vi "KE622x -- Set Current Range.vi"(0 "Resource In":refnum<visa-resource-name>, 1 "Check For SCPI Errors? (T)":bool=TRUE, 7 "Current Range In":T1, 11 "error in (no error)":errorcluster, 12 "Read Back Set Values? (T)":bool=TRUE) -> (4 "Resource Out (dupl)":refnum<visa-resource-name>, 8 "Current Range Out":T1, 15 "error out":errorcluster)   [LabVIEW 2020, in "Keithley 622x.lvlib"]
doc: "Allows the user to either auto-select the current range based on the current level, or manually specify a range."
uses:
  Keithley 622x.lvlib
  Typedefs/KE622x -- Current Ranges.ctl
  C/Program Files/National Instruments/LabVIEW 2021/instr.lib/Keithley 622x LV 2009/Configure/Source/Typedefs/KE622x -- Current Range.ctl
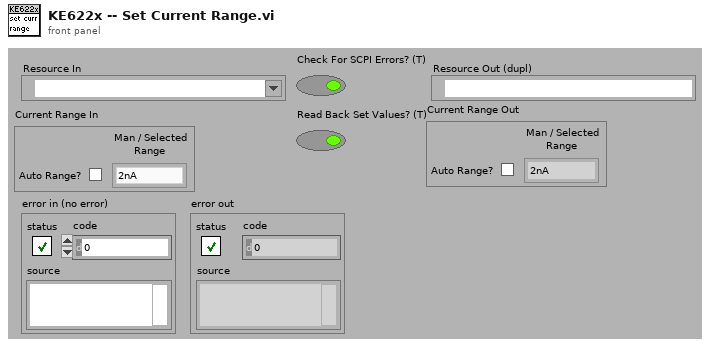
[diagram p1: front panel]
types:
  T1 = typedef "Keithley 622x.lvlib/KE622x -- Current Range.ctl" = cluster{"Auto Range?":bool, "Man / Selected\nRange":T2}
  T2 = typedef "Keithley 622x.lvlib/KE622x -- Current Ranges.ctl" = enum16{"2nA", "20nA", "200nA", "2uA", "20uA", "200uA", "2mA", "20mA", "100mA"}
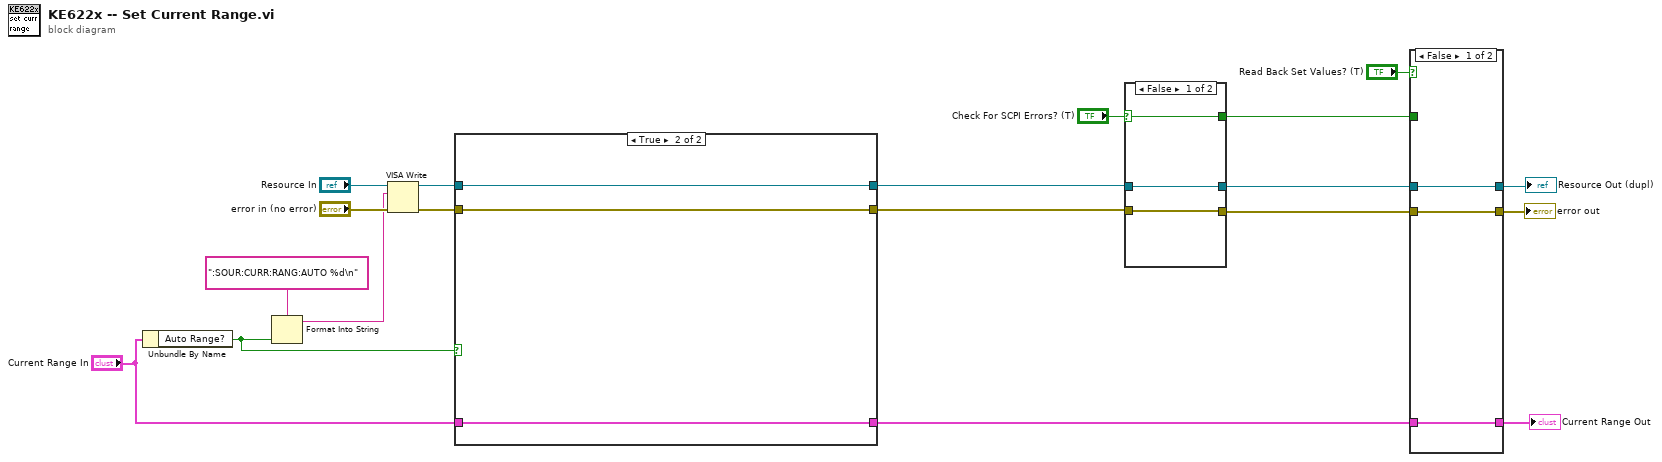
[diagram p0: block diagram]
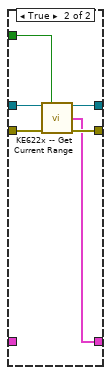
[diagram p2: hidden frame]
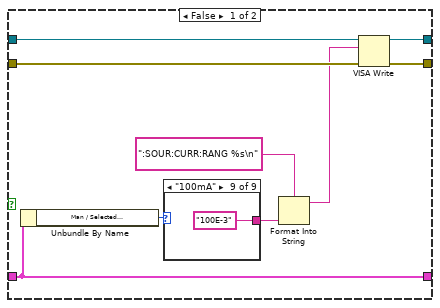
[diagram p3: hidden frame]
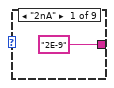
[diagram p4: hidden frame]
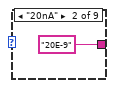
[diagram p5: hidden frame]
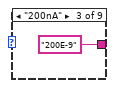
[diagram p6: hidden frame]
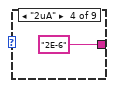
[diagram p7: hidden frame]
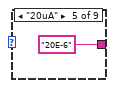
[diagram p8: hidden frame]
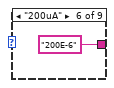
[diagram p9: hidden frame]
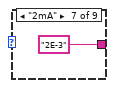
[diagram p10: hidden frame]
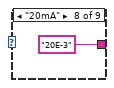
[diagram p11: hidden frame]
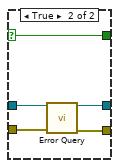
[diagram p12: hidden frame]
diagram:
  n1 = Unbundle By Name("Current Range In") -> ("Auto Range?"=w12:bool)
  n2 = Format Into String(format string=":SOUR:CURR:RANG:AUTO %d\n", w12) -> (resulting string=w15:string)  [unwired: 2 in, 1 out]
  n3 = VISA Write(VISA resource name="Resource In", write buffer=w15, error in (no error)="error in (no error)") -> (VISA resource name out=w14:refnum<visa-resource-name>, error out=w13:errorcluster)  [unwired: 1 out]
  n4 = case shown="True" w12 {
    tunnel: w14 -> [w28 w40]
    tunnel: w13 -> [w27 w39]
    tunnel: "Current Range In" -> [w20 w38]
    tunnel: [w22 w39] -> w9
    tunnel: [w21 w40] -> w10
    tunnel: [w20 w38] -> w4
    frame False {
      n5 = Unbundle By Name(w20) -> ("Man / Selected\nRange"=w26:T2)
      n6 = case shown="\"100mA\"" w26 {
        tunnel: ["2E-9" "20E-9" "200E-9" "2E-6" "20E-6" "200E-6" "2E-3" "20E-3" "100E-3"] -> w24
        frame "2nA" {
        }
        frame "20nA" {
        }
        frame "200nA" {
        }
        frame "2uA" {
        }
        frame "20uA" {
        }
        frame "200uA" {
        }
        frame "2mA" {
        }
        frame "20mA" {
        }
        frame "100mA" {
        }
      }
      n7 = Format Into String(format string=":SOUR:CURR:RANG %s\n", w24) -> (resulting string=w23:string)  [unwired: 2 in, 1 out]
      n8 = VISA Write(VISA resource name=w28, write buffer=w23, error in (no error)=w27) -> (VISA resource name out=w21:refnum<visa-resource-name>, error out=w22:errorcluster)  [unwired: 1 out]
    }
    frame True {
    }
  }
  n9 = case shown="False" "Check For SCPI Errors? (T)" {
    selector: "Check For SCPI Errors? (T)" -> [w41 w44]
    tunnel: w10 -> [w43 w48]
    tunnel: w9 -> [w42 w47]
    tunnel: [w42 w46] -> w7
    tunnel: [w43 w45] -> w8
    tunnel: [w41 w44] -> w5
    frame False {
    }
    frame True {
      n10 = call "Error Query.vi"("VISA Resource In"=w48, "error in (no error)"=w47) -> ("VISA Resource Out (dupl)"=w45:refnum<visa-resource-name>, "error out"=w46:errorcluster)  [unwired: 10 in, 2 out]
    }
  }
  n11 = case shown="False" "Read Back Set Values? (T)" {
    tunnel: w8 -> [w50 w57]
    tunnel: w7 -> [w49 w56]
    tunnel: w5 -> [_ w55]
    tunnel: [w50 w54] -> w3
    tunnel: [w49 w53] -> w2
    tunnel: w4 -> [w51 _]
    tunnel: [w51 w52] -> w1
    frame False {
    }
    frame True {
      n12 = call "KE622x -- Get Current Range.vi"("Resource In"=w57, "Check For SCPI Errors? (T)"=w55, "error in (no error)"=w56) -> ("Resource Out (dupl)"=w54:refnum<visa-resource-name>, "Current Range"=w52:T1, "error out"=w53:errorcluster)  [unwired: 10 in]
    }
  }
  "Resource Out (dupl)" <- w3
  "error out" <- w2
  "Current Range Out" <- w1
